vi "Поиск названий и вывод в массив.vi"() -> ()   [LabVIEW 2021]
panel:
  out "Array":string[](array[string])
  out "appended array":i32[](array[numeric])
  out "concatenated string":string
  out "filenames":string[](array[string])
  in  "stop":bool
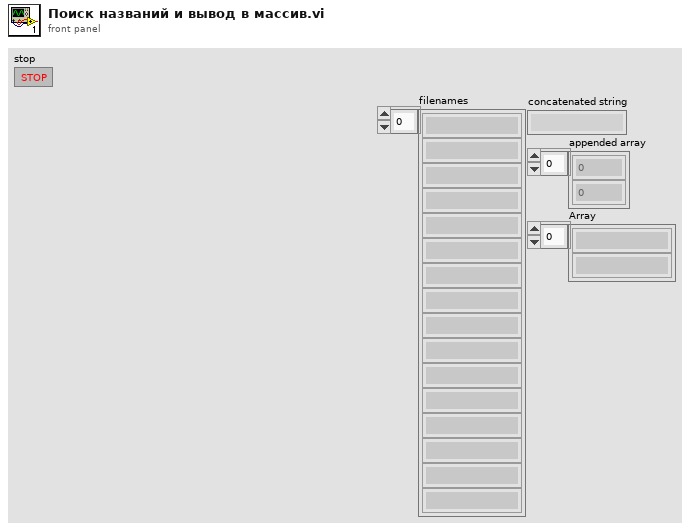
[diagram p1: front panel]
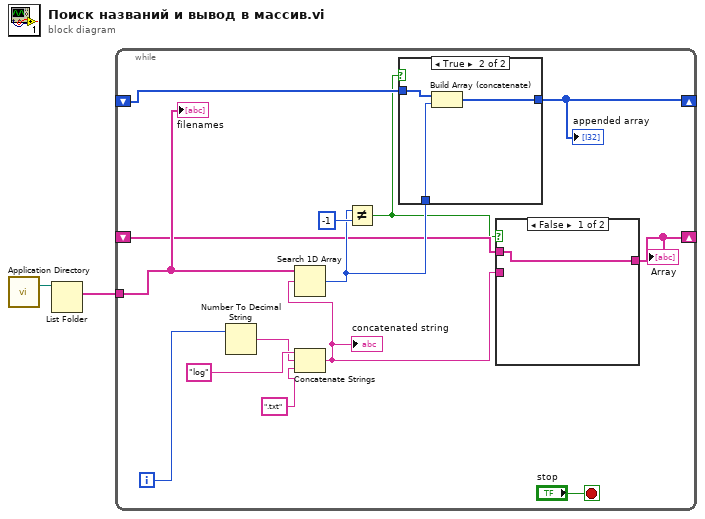
[diagram p0: block diagram]
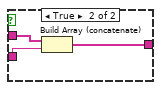
[diagram p2: hidden frame]
diagram:
  n1 = call <vilib>:"Application Directory.vi"() -> ("Application Directory"=w2:path)
  n2 = List Folder(path=w2) -> (filenames=w1:string[])  [unwired: 3 in, 3 out]
  n3 = while {
    tunnel: w1 -> [w11]
    shift-right: [w7] -> _
    shift-left: _ -> [w9]
    shift-right: [w6] -> _
    shift-left: _ -> [w5]
    i -> [w14]
    stop <- "stop" stop-if-true
    n4 = Number To Decimal String(number=w14) -> (decimal integer string=w12:string)  [unwired: 1 in]
    n5 = Concatenate Strings("log", w12, ".txt") -> (w3:string)
    "concatenated string" <- w3
    n6 = Search 1D Array(1D array=w11, element=w3) -> (index of element=w8:i32)  [unwired: 1 in]
    n7 = Not Equal?(x=w8, y=-1) -> (x != y?=w4:bool)
    n8 = case shown="True" w4 {
      tunnel: w9 -> [w21 w24]
      tunnel: [w21 w23] -> w7
      tunnel: w8 -> [_ w22]
      frame False {
      }
      frame True {
        n9 = Build Array (concatenate)(w24, w22) -> (w23:i32[])
      }
    }
    "appended array" <- w7
    n10 = case shown="False" w4 {
      tunnel: w5 -> [w17 w20]
      tunnel: [w17 w19] -> w6
      tunnel: w3 -> [_ w18]
      frame False {
      }
      frame True {
        n11 = Build Array (concatenate)(w20, w18) -> (w19:string[])
      }
    }
    "Array" <- w6
    "filenames" <- w11
  }
